vi "Exit In Place Element Array.vi"(0 "Diagram in":refnum<vi>, 5 "Elements":refnum<vi>[](array[refnum]), 7 "Outputs":refnum<vi>[](array[refnum]), 11 "error in (no error)":errorcluster) -> (4 "Diagram out":refnum<vi>, 6 "Array":refnum<vi>, 8 "Indices":refnum<vi>[][](array[refnum]), 10 "Outputs":refnum<vi>[](array[refnum]), 15 "error out":errorcluster)   [LabVIEW 2015, in "Scripting.lvlib"]
doc: "Exits the In Place Element Structure that owns <B>Diagram in</B>, supplying the structure's owning diagram at <B>Diagram out</B>.\n\n<B>Elements</B> are the terminals to wire to the Replace Array Subset node's element terminals.\n\n<B>Array</B> is the array output terminal of the Replace Array Subset node.\n\n<B>Indices</B> are the index output terminals of the Replace Array Subset node."
uses:
  Scripting.lvlib
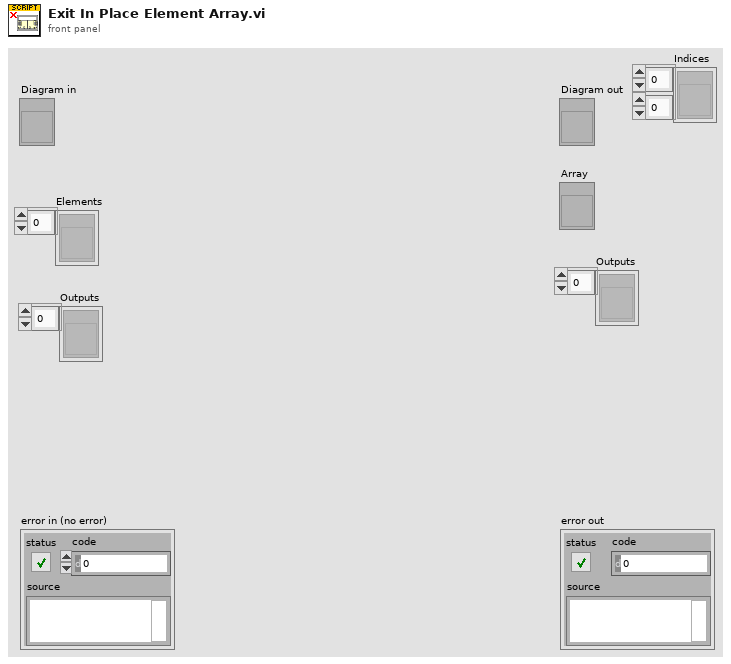
[diagram p1: front panel]
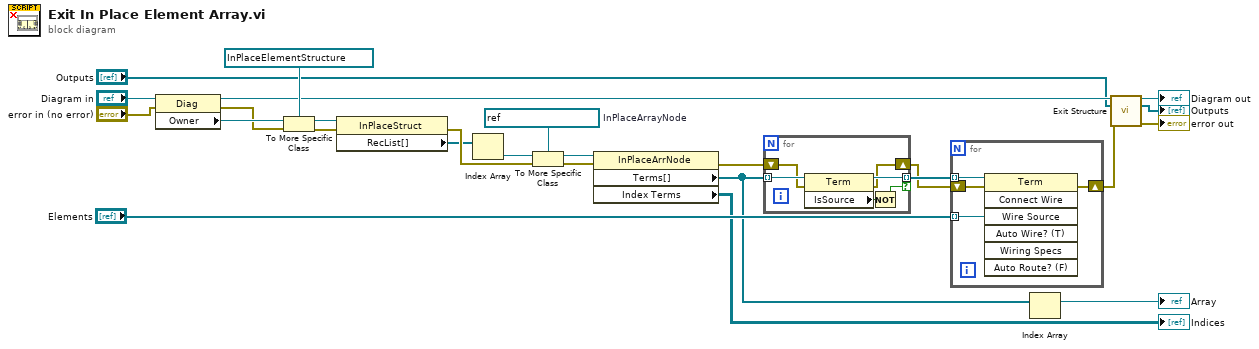
[diagram p0: block diagram]
diagram:
  w8 = refnum<vi> refnum  # InPlaceArrayNode
  n1 = property class="Diag"(reference="Diagram in", error in="error in (no error)") -> (reference out=w16:refnum<vi>, error out=w18:errorcluster, "Owner"=w26:refnum<vi>)
  n2 = To More Specific Class(target class=refnum<vi> refnum ("reference"), reference=w26, error in=w18) -> (specific class reference=w22:refnum<vi>, error out=w24:errorcluster)
  n3 = property class="InPlaceStruct"(reference=w22, error in=w24) -> (error out=w25:errorcluster, "RecList[]"=w23:refnum<vi>[])  [unwired: 1 out]
  n4 = Index Array(array=w23) -> (element=w10:refnum<vi>)  [unwired: 1 in]
  n5 = To More Specific Class(target class=w8, reference=w10, error in=w25) -> (specific class reference=w9:refnum<vi>, error out=w11:errorcluster)
  n6 = property class="InPlaceArrNode"(reference=w9, error in=w11) -> (error out=w3:errorcluster, "Terms[]"=w4:refnum<vi>[], "Index Terms"=→"Indices":refnum<vi>[][])  [unwired: 1 out]
  n7 = for {
    tunnel: w4 -> [w32] mode=indexing
    tunnel: [w31] -> w2 mode=indexing if=w29
    shift-right: [w27] -> w1
    shift-left: w3 -> [w28]
    n8 = property class="Term"(reference=w32, error in=w28) -> (reference out=w31:refnum<vi>, error out=w27:errorcluster, "IsSource"=w30:bool)
    n9 = Not(x=w30) -> (.not. x?=w29:bool)
  }
  n10 = for {
    tunnel: "Elements" -> [w35] mode=indexing
    shift-right: [w34] -> w17
    shift-left: w1 -> [w36]
    tunnel: w2 -> [w33] mode=indexing
    n11 = invoke class="Term" method="Connect Wire"(reference=w33, error in=w36, "Wire Source"=w35) -> (error out=w34:errorcluster)  [unwired: 4 in, 6 out]
  }
  n12 = Index Array(array=w4) -> (element=→"Array":refnum<vi>)  [unwired: 1 in]
  n13 = call "Exit Structure.vi"("Diagram in"=w16, "Outputs"="Outputs", "error in (no error)"=w17) -> ("Diagram out"=→"Diagram out":refnum<vi>, "Outputs"=→"Outputs":refnum<vi>[], "error out"=→"error out":errorcluster)  [unwired: 10 in]
